vi "Thermal Chamber Controller.vi"   [LabVIEW 2020]
uses:
  Thermal Chamber Controller/Thermal Chamber Controller.lvclass
  C:/Program Files (x86)/National Instruments/LabVIEW 2020/vi.lib/Astemes/Triarc Framework/Process/Process.lvclass
  C:/Program Files (x86)/National Instruments/LabVIEW 2020/vi.lib/Astemes/Triarc Framework/View/View.lvclass
  Thermal Chamber Controller/Private/Heater State.ctl
  <vilib>/Astemes/Triarc Framework/Process/Process.lvclass/Process.ctl
  <vilib>/Astemes/Triarc Framework/View/View.lvclass/View.ctl
  <vilib>/Astemes/Triarc Framework/Process/Protected/Messaging/Enqueue Message.vi
  <vilib>/Astemes/Triarc Framework/View/Public/Get View VI Reference.vi
  <vilib>/Astemes/Triarc Framework/Process/Public/Lifecycle/Get Lifecycle State.vi
  <vilib>/Astemes/Triarc Framework/Process/Private/SubVIs/Wait for finish.vi
  <vilib>/Astemes/Triarc Framework/Process/Private/SubVIs/Set Lifecycle State.vi
  <vilib>/Astemes/Triarc Framework/Process/Private/SubVIs/Handle Debug Data.vi
  <vilib>/Astemes/Triarc Framework/Process/Protected/Messaging/Request Message.vi
  <vilib>/Utility/error.llb/Clear Errors.vi
  <vilib>/Utility/High Resolution Relative Seconds.vi
  <vilib>/Astemes/Triarc Framework/Process/Private/SubVIs/Enqueue Request Message.vi
  <vilib>/Astemes/Triarc Framework/View/View.lvclass
  <vilib>/Utility/error.llb/Error Cluster From Error Code.vi
  <vilib>/Astemes/Triarc Framework/Process/Private/SubVIs/Wait for Response Message.vi
  <vilib>/Astemes/Triarc Framework/Process/Process.lvclass
types:
  T1 = typedef "Thermal Chamber Controller.lvclass/Heater State.ctl" = enum16{"Heater Disabled", "Heater Enabled"}
  T2 = typedef "Thermal Chamber Controller.lvclass/Chamber State.ctl" = cluster{"Actual Temperature":dbl, "Temperature Set Point":dbl, "Temperature Ramp Rate":dbl, "Heater State":T1}
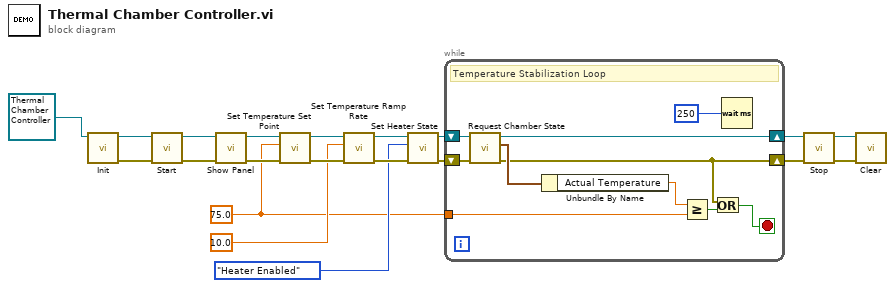
[diagram p0: block diagram]
diagram:
  w1 = 75.0 ("Temperature Set Point")
  n1 = call-dynamic "Init.vi"("View In"=refnum<class "Thermal Chamber Controller.lvclass"> refnum ("Thermal Chamber Controller.lvclass")) -> ("error out"=w19:errorcluster, "View Out"=w20:refnum<class "Thermal Chamber Controller.lvclass">)  [unwired: 9 in]
  n2 = call <vilib>:"Start.vi"("error in (no error)"=w19, "Process In"=w20) -> ("error out"=w18:errorcluster, "Process Out"=w13:refnum<class "Thermal Chamber Controller.lvclass">)  [unwired: 7 in, 1 out]
  n3 = call <vilib>:"Show Panel.vi"("error in (no error)"=w18, "View In"=w13) -> ("error out"=w14:errorcluster, "View Out"=w11:refnum<class "Thermal Chamber Controller.lvclass">)  [unwired: 8 in]
  n4 = call "Set Temperature Set Point.vi"("error in (no error)"=w14, "Temperature Set Point"=w1, "Thermal Chamber Controller In"=w11) -> ("error out"=w12:errorcluster, "Thermal Chamber Controller Out"=w9:refnum<class "Thermal Chamber Controller.lvclass">)  [unwired: 7 in]
  n5 = call "Set Temperature Ramp Rate.vi"("error in (no error)"=w12, "Temperature Ramp Rate [degC/s]"=10.0, "Thermal Chamber Controller In"=w9) -> ("error out"=w10:errorcluster, "Thermal Chamber Controller Out"=w6:refnum<class "Thermal Chamber Controller.lvclass">)  [unwired: 7 in]
  n6 = call "Set Heater State.vi"("error in (no error)"=w10, "Heater State"=Heater_State."Heater Enabled", "Thermal Chamber Controller In"=w6) -> ("error out"=w7:errorcluster, "Thermal Chamber Controller Out"=w3:refnum<class "Thermal Chamber Controller.lvclass">)  [unwired: 7 in]
  n7 = while {
    shift-right: [w25] -> w4
    shift-left: w7 -> [w30]
    shift-right: [w28] -> w2
    shift-left: w3 -> [w29]
    tunnel: w1 -> [w22]
    stop <- w26 stop-if-true
    # "Temperature Stabilization Loop"
    n8 = call "Request Chamber State.vi"("error in (no error)"=w30, "Thermal Chamber Controller In"=w29) -> ("error out"=w25:errorcluster, "Chamber Status Reply Payload"=w27:T2, "Thermal Chamber Controller Out"=w28:refnum<class "Thermal Chamber Controller.lvclass">)  [unwired: 6 in, 1 out]
    n9 = Unbundle By Name(w27) -> ("Actual Temperature"=w23:dbl)
    n10 = Greater Or Equal?(x=w23, y=w22) -> (x >= y?=w21:bool)
    n11 = Or(x=w25, y=w21) -> (x .or. y?=w26:bool)
    n12 = Wait (ms)(milliseconds to wait=u32 250) -> ()  [unwired: 1 out]
  }
  n13 = call <vilib>:"Stop.vi"("error in (no error)"=w4, "Process In"=w2) -> ("error out"=w16:errorcluster, "Process Out"=w17:refnum<class "Thermal Chamber Controller.lvclass">)  [unwired: 7 in, 1 out]
  n14 = call-dynamic "Clear.vi"("error in (no error)"=w16, "View In"=w17) -> ()  [unwired: 9 in, 1 out]
